vi "Write Template Library File Path.vi"(10 "Template Library File Path":path, 11 "_Template in":refnum<class "_Template.lvclass">) -> (3 "_Template out":refnum<class "_Template.lvclass">)   [LabVIEW 2020, in "_Template.lvlib" / "_Template.lvclass"]
uses:
  _Template.lvclass
  _Template.lvclass/_Template.ctl
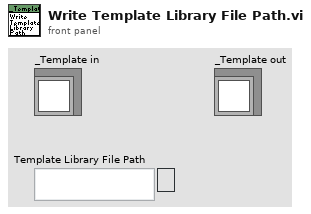
[diagram p1: front panel]
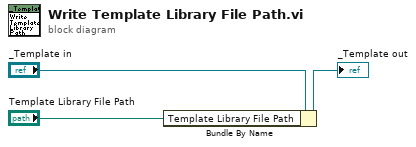
[diagram p0: block diagram]
diagram:
  n1 = Bundle By Name(cluster="_Template in", "Template Library File Path"="Template Library File Path") -> (→"_Template out":refnum<class "_Template.lvclass">)
